vi "Sub_Sharp_Vorne_seitlich.vi"(10 "rechts vorne":dbl, 11 "links vorne":dbl) -> (2 "lower than 5?":bool, 3 "IR Regelung Seite":dbl)   [LabVIEW 2016]
uses:
  <vilib>/addons/control/pid/pid.llb/PID (DBL).vi
  <vilib>/addons/control/pid/NI_PID_pid.lvlib
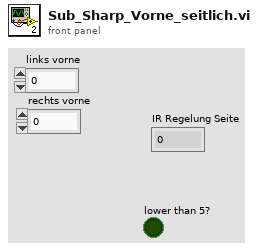
[diagram p1: front panel]
types:
  T1 = cluster{"proportional gain (Kc)":dbl, "integral time (Ti, min)":dbl, "derivative time (Td, min)":dbl}
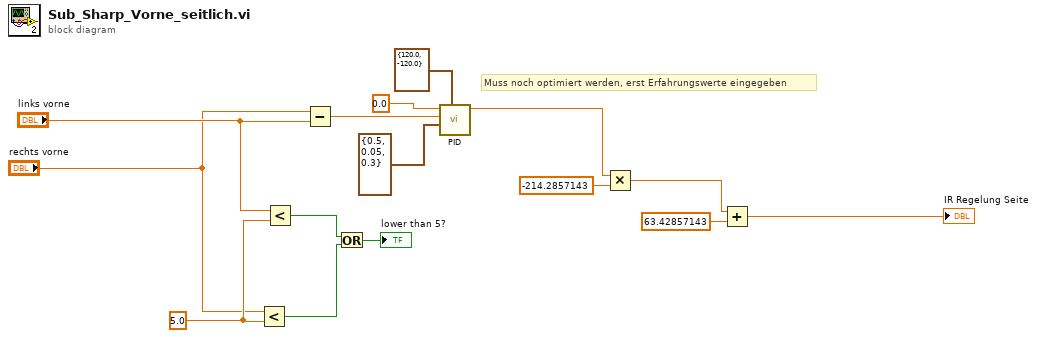
[diagram p0: block diagram]
diagram:
  w4 = 5.0 ("y")
  # "Muss noch optimiert werden, erst Erfahrungswerte eingegeben"
  n1 = Less?(x="rechts vorne", y=w4) -> (x < y?=w5:bool)
  n2 = Less?(x="links vorne", y=w4) -> (x < y?=w14:bool)
  n3 = Subtract(x="rechts vorne", y="links vorne") -> (x-y=w6:dbl)
  n4 = Or(x=w14, y=w5) -> (x .or. y?=→"lower than 5?":bool)
  n5 = call-poly <vilib>:"PID.vi"("output range"=cluster{"output high":dbl, "output low":dbl} {"output high"=120.0, "output low"=-120.0}, "PID gains"=T1 {"proportional gain (Kc)"=0.5, "integral time (Ti, min)"=0.05, "derivative time (Td, min)"=0.3}, "process variable"=w6, "setpoint"=0.0) -> ("output"=w13:dbl)  [unwired: 6 in, 1 out]
  n6 = Multiply(x=w13, y=-214.2857143) -> (x*y=w12:dbl)
  n7 = Add(x=w12, y=63.42857143) -> (x+y=→"IR Regelung Seite":dbl)
